vi "Add_New_Device.vi"(7 "LabVIEW Web Service Request":refnum<class "Web Request.lvclass">) -> ()   [LabVIEW 2016]
uses:
  <vilib>/wsapi/Web Request.lvclass
  Device Info.ctl
  Inventory FGV Command.ctl
panel:
  # "Use the Web Service Request input terminal to call the VIs on the Web Services palette. Do not remove it from the connector pane unless you don't need access to the palette."
  # "Each additional control wired to the connector pane will be available as an input in the URL. To include an indicator in terminal-mode output (the default setting), it must also be wired to the connector pane."
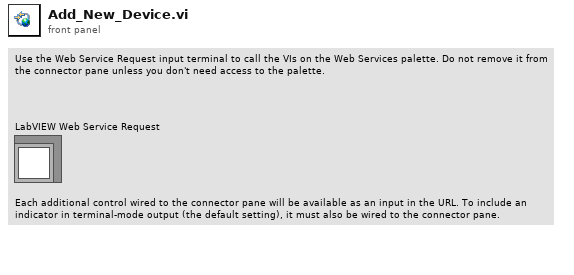
[diagram p1: front panel]
types:
  T1 = typedef "Inventory FGV Command.ctl" = enum16{"Load Items", "Check Status", "Return Items", "Check Out Items", "Add New Item", "Get All Items", "Remove Item", "Search"}
  T2 = typedef "Device Info.ctl" = cluster{"Model Number":string, "Identifier":string, "Available?":bool, "Owner":string, "Owner Email":string, "Last Activity Date":string, "Loan Purpose":string, "Department":string, "Notes":string, "Serial Number":string}
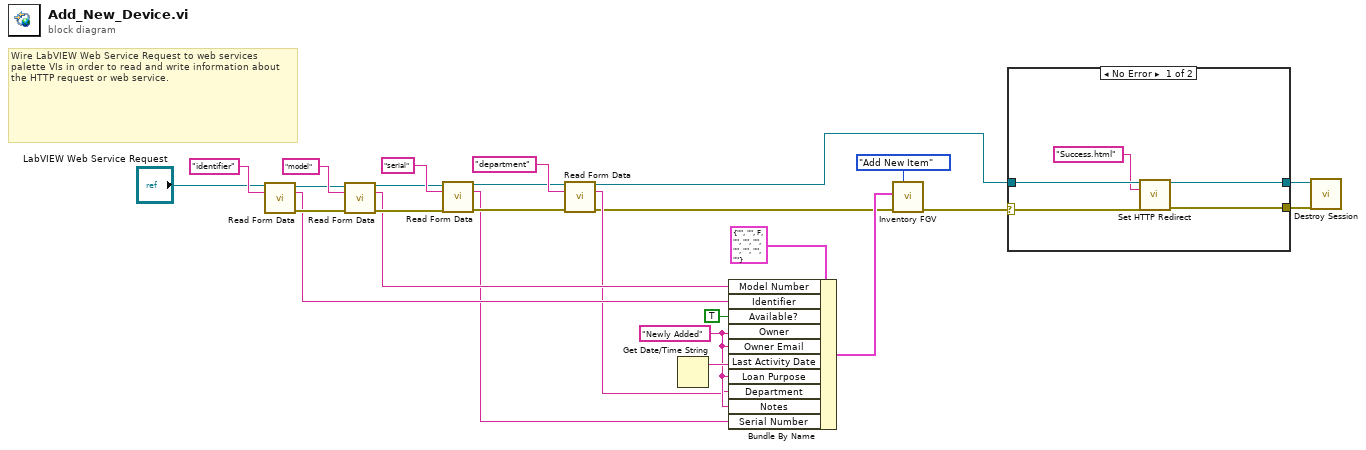
[diagram p0: block diagram]
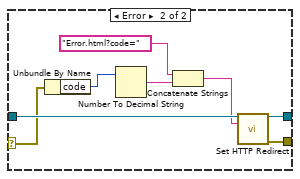
[diagram p2: hidden frame]
diagram:
  w10 = "Newly Added" ("Owner")
  # "Wire LabVIEW Web Service Request to web services palette VIs in order to read and write information about the HTTP request or web service."
  n1 = call <vilib>:"Read Form Data.vi"("LabVIEW Web Service Request"="LabVIEW Web Service Request", "key"="identifier") -> ("LabVIEW Web Service Request out"=w23:refnum<class "Web Request.lvclass">, "value"=w13:string, "error out"=w18:errorcluster)  [unwired: 10 in, 1 out]
  n2 = call <vilib>:"Read Form Data.vi"("LabVIEW Web Service Request"=w23, "key"="model", "error in (no error)"=w18) -> ("LabVIEW Web Service Request out"=w21:refnum<class "Web Request.lvclass">, "value"=w14:string, "error out"=w17:errorcluster)  [unwired: 9 in, 1 out]
  n3 = call <vilib>:"Read Form Data.vi"("LabVIEW Web Service Request"=w21, "key"="serial", "error in (no error)"=w17) -> ("LabVIEW Web Service Request out"=w19:refnum<class "Web Request.lvclass">, "value"=w8:string, "error out"=w16:errorcluster)  [unwired: 9 in, 1 out]
  n4 = call <vilib>:"Read Form Data.vi"("LabVIEW Web Service Request"=w19, "key"="department", "error in (no error)"=w16) -> ("LabVIEW Web Service Request out"=w3:refnum<class "Web Request.lvclass">, "value"=w9:string, "error out"=w5:errorcluster)  [unwired: 9 in, 1 out]
  n5 = Get Date/Time String() -> (date string=w11:string)  [unwired: 3 in, 1 out]
  n6 = Bundle By Name(cluster=T2 {"Model Number"="", "Identifier"="", "Available?"=FALSE, "Owner"="", "Owner Email"="", "Last Activity Date"="", "Loan Purpose"="", "Department"="", "Notes"="", "Serial Number"=""} ("Device"), "Model Number"=w14, "Identifier"=w13, "Available?"=TRUE, "Owner"=w10, "Owner Email"=w10, "Last Activity Date"=w11, "Loan Purpose"=w10, "Department"=w9, "Notes"=w10, "Serial Number"=w8) -> (w6:T2)
  n7 = call "Inventory FGV.vi"("error in"=w5, "Device Info"=w6, "Command"=Inventory_FGV_Command."Add New Item") -> ("error out"=w4:errorcluster)  [unwired: 5 in, 2 out]
  n8 = case shown="No Error" w4 {
    selector: w4 -> [w31 w38]
    tunnel: w3 -> [w30 w39]
    tunnel: [w29 w33] -> w2
    tunnel: [w28 w32] -> w1
    frame No Error {
      n9 = call <vilib>:"Set HTTP Redirect.vi"("LabVIEW Web Service Request"=w30, "redirect URL"="Success.html", "error in (no error)"=w31) -> ("LabVIEW Web Service Request out"=w29:refnum<class "Web Request.lvclass">, "error out"=w28:errorcluster)  [unwired: 11 in]
    }
    frame Error {
      n10 = Unbundle By Name(w38) -> ("code"=w36:i32)
      n11 = Number To Decimal String(number=w36) -> (decimal integer string=w35:string)  [unwired: 1 in]
      n12 = Concatenate Strings("Error.html?code=", w35) -> (w34:string)
      n13 = call <vilib>:"Set HTTP Redirect.vi"("LabVIEW Web Service Request"=w39, "redirect URL"=w34) -> ("LabVIEW Web Service Request out"=w33:refnum<class "Web Request.lvclass">, "error out"=w32:errorcluster)  [unwired: 12 in]
    }
  }
  n14 = call <vilib>:"Destroy Session.vi"("LabVIEW Web Service Request"=w2, "error in (no error)"=w1) -> ()  [unwired: 12 in, 2 out]
